vi "New (Element).vi"(6 "include descendants? (T)":bool, 7 "scope type (VI)":enum16{"VI", "Library", "Class"}(ring), 10 "match behavior (keep)":T1, 11 "scope name (\"\")":string) -> (3 "basic scope":refnum<class "Basic.lvclass">)   [LabVIEW 2018, in "Logging.lvlib" / "Basic.lvclass"]
uses:
  Basic.lvclass
  Match Behavior.ctl
  Aggregation Method.ctl
  Logging.lvlib
panel:
  # "Connector Pane"
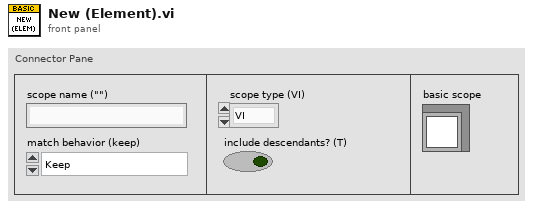
[diagram p1: front panel]
types:
  T1 = typedef "Logging.lvlib/Match Behavior.ctl" = enum16{"Keep", "Discard"}
  T2 = typedef "Logging.lvlib/Aggregation Method.ctl" = enum16{"Any", "Only", "All", "None"}
  T3 = cluster{"Name":string, "Type":enum16{"VI", "Library", "Class"}, "Include Descendants?":bool}[]
  T4 = cluster{"Name":string, "Type":enum16{"VI", "Library", "Class"}, "Include Descendants?":bool}
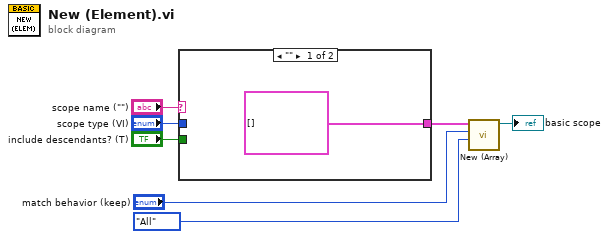
[diagram p0: block diagram]
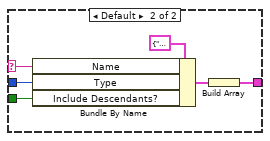
[diagram p2: hidden frame]
diagram:
  n1 = case shown="\"\"" "scope name (\"\")" {
    selector: "scope name (\"\")" -> [_ w13]
    tunnel: "scope type (VI)" -> [_ w12]
    tunnel: "include descendants? (T)" -> [_ w11]
    tunnel: [T3 [] w9] -> w4
    frame "" {
    }
    frame Default {
      n2 = Bundle By Name(cluster=T4 {"Name"="", "Type"=enum."VI", "Include Descendants?"=FALSE} ("scope info"), "Name"=w13, "Type"=w12, "Include Descendants?"=w11) -> (w10:T4)
      n3 = Build Array(w10) -> (w9:T3)
    }
  }
  n4 = call "New (Array).vi"("aggregation method (all)"=Aggregation_Method."All", "match behavior (keep)"="match behavior (keep)", "scope info"=w4) -> ("basic scope"=→"basic scope":refnum<class "Basic.lvclass">)  [unwired: 8 in]
